vi "DEBUG_VERBOSE.vi"(10 "argv":string[](array[string]), 11 "args":u8) -> ()   [LabVIEW 2011]
uses:
  <vilib>/Rock Robotics/WPI/DriverStation/WPI_DriverStationStatusErrorCache.ctl
  Auto_Conf.vi
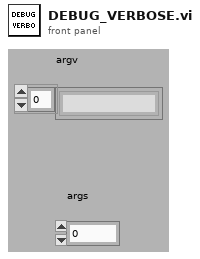
[diagram p1: front panel]
types:
  T1 = typedef "WPI_DriverStationStatusErrorCache.ctl" = enum16{"Get", "Set"}
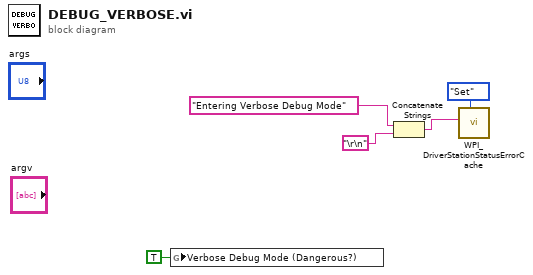
[diagram p0: block diagram]
diagram:
  n1 = global write "Auto_Conf.vi" "Verbose Debug Mode (Dangerous?)"(TRUE ("Verbose Debug Mode (Dangerous?)")) -> ()
  n2 = Concatenate Strings("Entering Verbose Debug Mode" ("string"), "\r\n") -> (w3:string)
  n3 = call <vilib>:"WPI_DriverStationStatusErrorCache.vi"("StatusErrorCacheOp"=WPI_DriverStationStatusErrorCache."Set", "Error String"=w3) -> ()  [unwired: 10 out]
